vi "Write Log.vi"(6 "Auto Stats":T1, 9 "OEE in":T3, 10 "output cluster":cluster{"GoodCount":u32, "RejectCount":u32}, 11 "refnum out":refnum<file>) -> ()   [LabVIEW 2021]
uses:
  support/Controls/Auto Stats.ctl
  RT/Controls/Auto Times.ctl
panel:
  out "error out":errorcluster
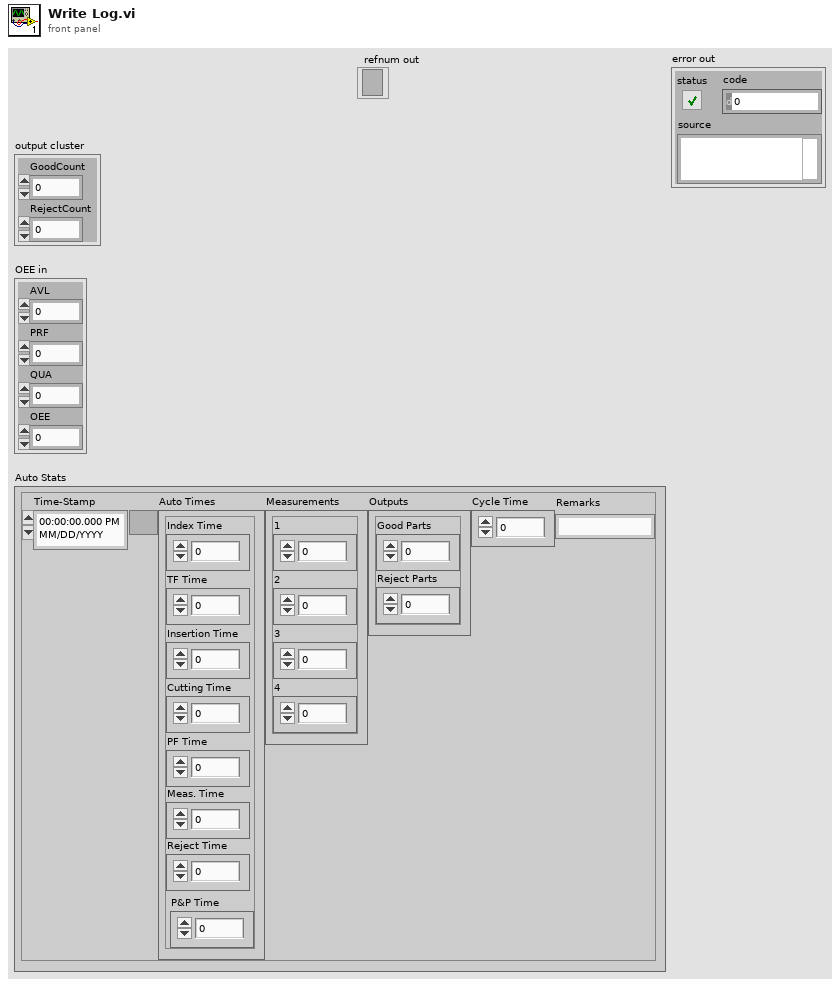
[diagram p1: front panel]
types:
  T1 = typedef "Auto Stats.ctl" = cluster{"Time-Stamp":timestamp, "Auto Times":T2, "Measurements":cluster{"1":dbl, "2":dbl, "3":dbl, "4":dbl}, "Outputs":cluster{"Good Parts":u32, "Reject Parts":u32}, "Cycle Time":dbl, "Remarks":string}
  T2 = typedef "Auto Times.ctl" = cluster{"Index Time":u32, "TF Time":u32, "Insertion Time":u32, "Cutting Time":u32, "PF Time":u32, "Meas. Time":u32, "Reject Time":u32, "P&P Time":u32}
  T3 = cluster{"AVL":dbl, "PRF":dbl, "QUA":dbl, "OEE":dbl}
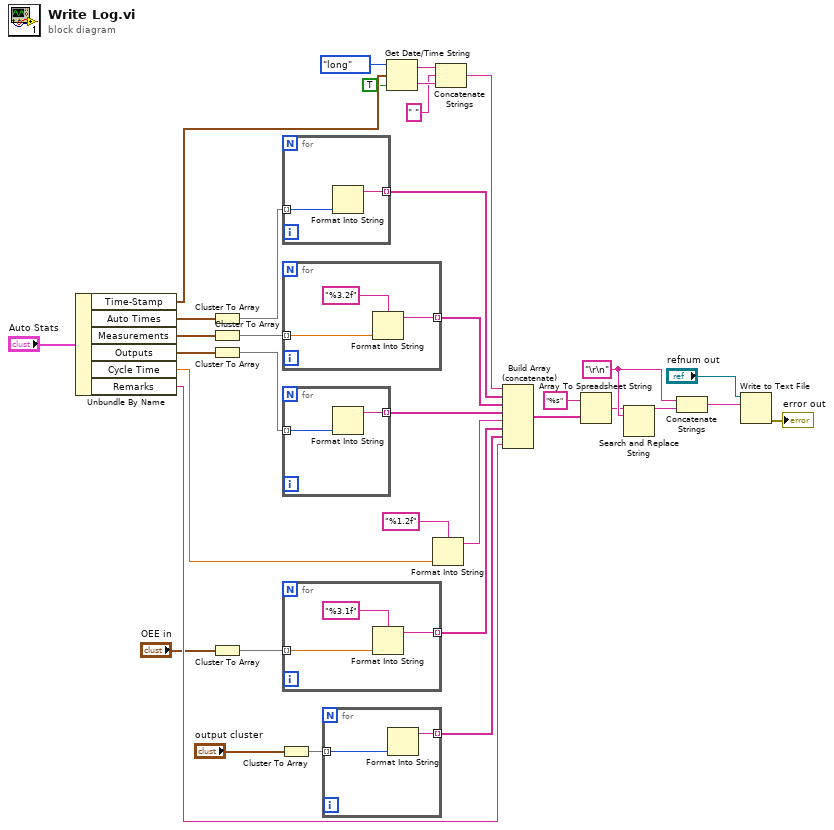
[diagram p0: block diagram]
diagram:
  w6 = "\r\n" ("replace string (\"\")")
  n1 = Unbundle By Name("Auto Stats") -> ("Time-Stamp"=w10:timestamp, "Auto Times"=w15:T2, "Measurements"=w19:cluster{"1":dbl, "2":dbl, "3":dbl, "4":dbl}, "Outputs"=w22:cluster{"Good Parts":u32, "Reject Parts":u32}, "Cycle Time"=w26:dbl, "Remarks"=w34:string)
  n2 = Cluster To Array(cluster=w15) -> (array=w16:u32[])
  n3 = Cluster To Array(cluster=w19) -> (array=w20:dbl[])
  n4 = Cluster To Array(cluster=w22) -> (array=w23:u32[])
  n5 = Cluster To Array(cluster="OEE in") -> (array=w29:dbl[])
  n6 = Cluster To Array(cluster="output cluster") -> (array=w32:u32[])
  n7 = for {
    tunnel: w16 -> [w37] mode=indexing
    tunnel: [w36] -> w18 mode=indexing
    n8 = Format Into String(w37) -> (resulting string=w36:string)  [unwired: 3 in, 1 out]
  }
  n9 = for {
    tunnel: w20 -> [w40] mode=indexing
    tunnel: [w39] -> w21 mode=indexing
    n10 = Format Into String(format string="%3.2f", w40) -> (resulting string=w39:string)  [unwired: 2 in, 1 out]
  }
  n11 = for {
    tunnel: w23 -> [w42] mode=indexing
    tunnel: [w41] -> w24 mode=indexing
    n12 = Format Into String(w42) -> (resulting string=w41:string)  [unwired: 3 in, 1 out]
  }
  n13 = for {
    tunnel: w29 -> [w45] mode=indexing
    tunnel: [w44] -> w30 mode=indexing
    n14 = Format Into String(format string="%3.1f", w45) -> (resulting string=w44:string)  [unwired: 2 in, 1 out]
  }
  n15 = for {
    tunnel: w32 -> [w47] mode=indexing
    tunnel: [w46] -> w33 mode=indexing
    n16 = Format Into String(w47) -> (resulting string=w46:string)  [unwired: 3 in, 1 out]
  }
  n17 = Get Date/Time String(date format (0)=enum16{"short", "long", "abbreviated"}."long", seconds (now)=w10, want seconds? (F)=TRUE) -> (date string=w12:string, time string=w14:string)
  n18 = Format Into String(format string="%1.2f", w26) -> (resulting string=w27:string)  [unwired: 2 in, 1 out]
  n19 = Concatenate Strings(w12, " " ("string"), w14) -> (w17:string)
  n20 = Build Array (concatenate)(w17, w18, w21, w24, w27, w30, w33, w34) -> (w35:string[])
  n21 = Array To Spreadsheet String(array=w35, 3:"%s" ("format string")) -> (spreadsheet string=w5:string)  [unwired: 1 in]
  n22 = Search and Replace String(input string=w5, search string=w6) -> (result string=w7:string)  [unwired: 6 in, 3 out]
  n23 = Concatenate Strings(w6, w7) -> (w8:string)
  n24 = Write to Text File(file (use dialog)="refnum out", text=w8) -> (error out=→"error out":errorcluster)  [unwired: 2 in, 2 out]
